vi "SwitchGratingPopup.vi"(7 "Monochromator in":T1={"Type"=enum."Oriel", "Wavelength (nm)"=0.0, "Wavelength (nm)"="", "Grating, gr/mm"=0, "Grating mode"=enum."IR", "Spectrum mode"={"Spectrum mode?"=FALSE, "Start wavelength (nm)"=0.0, "End wavelength (nm)"=0.0, "Wavelength step (nm)"=0.0, "Wavelength array"=[], "array index"=0}, "VISA"={"delay before read (ms)"=0, "Mono 1"={"Enable Termination Char (T)"=FALSE, "timeout (msec)"=0, "Resource name"="", "baud rate"=0, "data bits"=0, "parity"=0, "stop bits"=0, "flow control"=0}, "Mono 2"={"Enable Termination Char (T)"=FALSE, "timeout (msec)"=0, "Resource name"="", "baud rate"=0, "data bits"=0, "parity"=0, "stop bits"=0, "flow control"=0}}} {"VISA"."Mono 2"."flow control" items=["None"=0, "XON/XOFF"=1, "RTS/CTS"=2, "DTR/DSR"=4]; "VISA"."Mono 2"."stop bits" items=["None"=0, "XON/XOFF"=1, "RTS/CTS"=2, "DTR/DSR"=4]; "VISA"."Mono 2"."parity" items=["1.0"=10, "1.5"=15, "2.0"=20]; "VISA"."Mono 1"."flow control" items=["None"=0, "XON/XOFF"=1, "RTS/CTS"=2, "DTR/DSR"=4]; "VISA"."Mono 1"."stop bits" items=["None"=0, "XON/XOFF"=1, "RTS/CTS"=2, "DTR/DSR"=4]; "VISA"."Mono 1"."parity" items=["1.0"=10, "1.5"=15, "2.0"=20]; "Grating, gr/mm" items=["2400", "1800", "1200", "600", "300", "150"]}, 8 "error in (no error)":errorcluster, 11 "New wavelength (nm)":dbl) -> (0 "error out":errorcluster, 3 "New wavelength (nm)":dbl, 5 "Monochromator out":T1={"Type"=enum."Oriel", "Wavelength (nm)"=0.0, "Wavelength (nm)"="", "Grating, gr/mm"=0, "Grating mode"=enum."IR", "Spectrum mode"={"Spectrum mode?"=FALSE, "Start wavelength (nm)"=0.0, "End wavelength (nm)"=0.0, "Wavelength step (nm)"=0.0, "Wavelength array"=[], "array index"=0}, "VISA"={"delay before read (ms)"=0, "Mono 1"={"Enable Termination Char (T)"=FALSE, "timeout (msec)"=0, "Resource name"="", "baud rate"=0, "data bits"=0, "parity"=0, "stop bits"=0, "flow control"=0}, "Mono 2"={"Enable Termination Char (T)"=FALSE, "timeout (msec)"=0, "Resource name"="", "baud rate"=0, "data bits"=0, "parity"=0, "stop bits"=0, "flow control"=0}}} {"VISA"."Mono 2"."flow control" items=["None"=0, "XON/XOFF"=1, "RTS/CTS"=2, "DTR/DSR"=4]; "VISA"."Mono 2"."stop bits" items=["None"=0, "XON/XOFF"=1, "RTS/CTS"=2, "DTR/DSR"=4]; "VISA"."Mono 2"."parity" items=["1.0"=10, "1.5"=15, "2.0"=20]; "VISA"."Mono 1"."flow control" items=["None"=0, "XON/XOFF"=1, "RTS/CTS"=2, "DTR/DSR"=4]; "VISA"."Mono 1"."stop bits" items=["None"=0, "XON/XOFF"=1, "RTS/CTS"=2, "DTR/DSR"=4]; "VISA"."Mono 1"."parity" items=["1.0"=10, "1.5"=15, "2.0"=20]; "Grating, gr/mm" items=["2400", "1800", "1200", "600", "300", "150"]})   [LabVIEW 2017]
uses:
  Controls/Params.ctl
  Controls/Grating.ctl
  Controls/VISA parameters.ctl
  Monochromator.lvlib
  Serial comms/Serial comms.lvlib
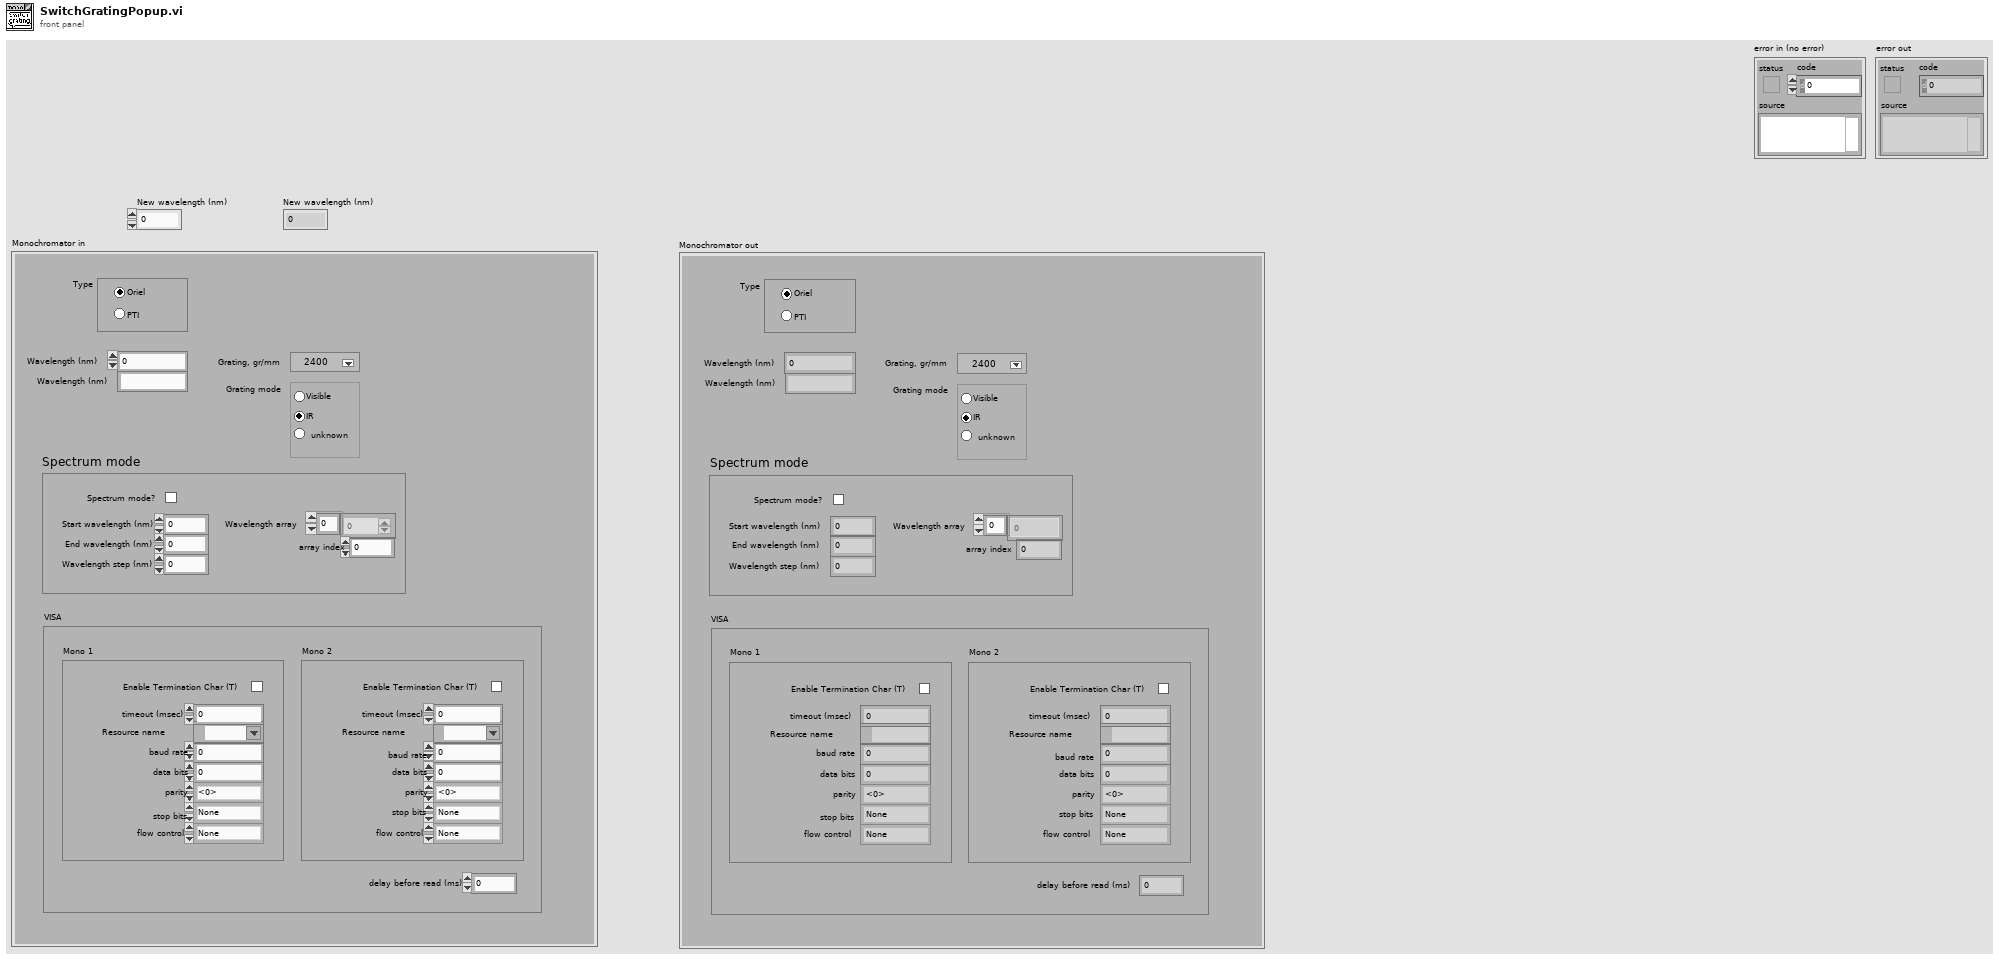
[diagram p1: front panel]
types:
  T1 = typedef "Monochromator.lvlib/Params.ctl" = cluster{"Type":enum32{"Oriel", "PTI"}, "Wavelength (nm)":dbl, "Wavelength (nm)":string, "Grating, gr/mm":u16, "Grating mode":T2, "Spectrum mode":cluster{"Spectrum mode?":bool, "Start wavelength (nm)":dbl, "End wavelength (nm)":dbl, "Wavelength step (nm)":dbl, "Wavelength array":dbl[], "array index":u32}, "VISA":cluster{"delay before read (ms)":u32, "Mono 1":T3, "Mono 2":T3}}
  T2 = typedef "Monochromator.lvlib/Grating.ctl" = enum32{"unknown", "Visible", "IR"}
  T3 = typedef "Serial comms.lvlib/VISA parameters.ctl" = cluster{"Enable Termination Char (T)":bool, "timeout (msec)":u32, "Resource name":refnum<visa-resource-name>, "baud rate":u32, "data bits":u16, "parity":u16, "stop bits":u16, "flow control":u16}
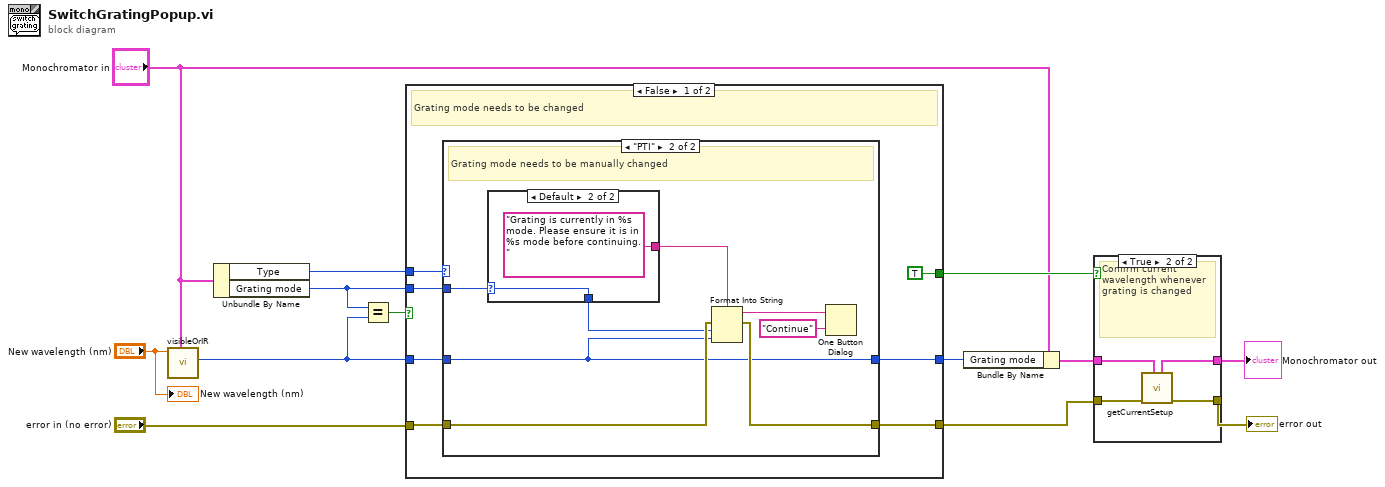
[diagram p0: block diagram]
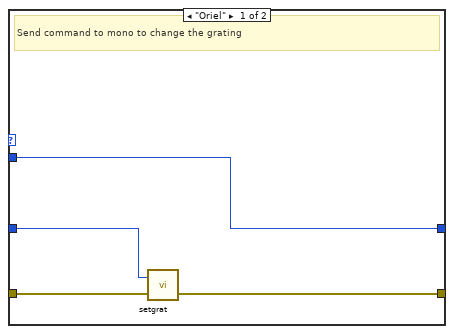
[diagram p3: hidden frame]
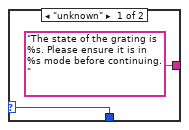
[diagram p4: hidden frame]
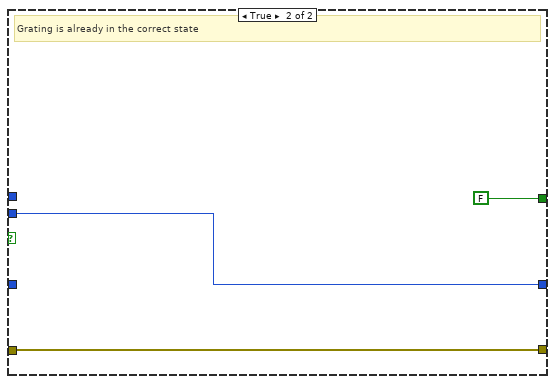
[diagram p5: hidden frame]
diagram:
  n1 = call "visibleOrIR.vi"("Monochromator"="Monochromator in", "Wavelength (nm)"="New wavelength (nm)") -> ("IR/visible"=w9:T2)  [unwired: 8 in, 1 out]
  n2 = Unbundle By Name("Monochromator in") -> ("Type"=w3:enum32{"Oriel", "PTI"}, "Grating mode"=w8:T2)
  n3 = Equal?(x=w8, y=w9) -> (x = y?=w13:bool)
  n4 = case shown="False" w13 {
    tunnel: w9 -> [w20 _]
    tunnel: w8 -> [w16 w39]
    tunnel: [w14 w39] -> w12
    tunnel: "error in (no error)" -> [w19 w38]
    tunnel: [w18 w38] -> w1
    tunnel: [TRUE FALSE] -> w7
    tunnel: w3 -> [w15 _]
    frame False {
      # "Grating mode needs to be changed"
      n5 = case shown="\"PTI\"" w15 {
        tunnel: w20 -> [w23 w25]
        tunnel: w19 -> [w24 w30]
        tunnel: [w22 w29] -> w18
        tunnel: w16 -> [w21 w28]
        tunnel: [w21 w25] -> w14
        frame "Oriel" {
          # "Send command to mono to change the grating"
          n6 = call "setgrat.vi"("error in (no error)"=w24, "Grating"=w23) -> ("error out"=w22:errorcluster)  [unwired: 1 in]
        }
        frame "PTI" {
          # "Grating mode needs to be manually changed"
          n7 = case shown="Default" w28 {
            selector: w28 -> [w34 w35]
            tunnel: ["The state of the grating is %s. Please ensure it is in %s mode before continuing." ("format string") "Grating is currently in %s mode. Please ensure it is in %s mode before continuing." ("format string")] -> w26
            tunnel: [w34 w35] -> w27
            frame "unknown" {
            }
            frame Default {
            }
          }
          n8 = Format Into String(format string=w26, error in=w30, w27, w25) -> (resulting string=w31:string, error out=w29:errorcluster)  [unwired: 1 in]
          n9 = One Button Dialog(message=w31, button name ("OK")="Continue") -> ()  [unwired: 1 out]
        }
      }
    }
    frame True {
      # "Grating is already in the correct state"
    }
  }
  n10 = Bundle By Name(cluster="Monochromator in", "Grating mode"=w12) -> (w6:T1)
  n11 = case shown="True" w7 {
    tunnel: w6 -> [w41 w45]
    tunnel: [w41 w44] -> w5
    tunnel: [w40 w42] -> w4
    tunnel: w1 -> [w40 w43]
    frame False {
    }
    frame True {
      # "Confirm current wavelength whenever grating is changed"
      n12 = call "getCurrentSetup.vi"("Monochromator in"=w45, "error in (no error)"=w43) -> ("error out"=w42:errorcluster, "Monochromator out"=w44:T1)  [unwired: 8 in]
    }
  }
  "error out" <- w4
  "Monochromator out" <- w5
  "New wavelength (nm)" <- "New wavelength (nm)"
